vi "AT Command Controller.vi"(2 "error in (no error)":errorcluster, 3 "Command List":T3(array[cluster]), 4 "Boolean Input":u32[](array[numeric])) -> (0 "error out":errorcluster)   [LabVIEW 2018]
uses:
  States.ctl
  Buttons.ctl
  Swerve Drive/Vision Mode.ctl
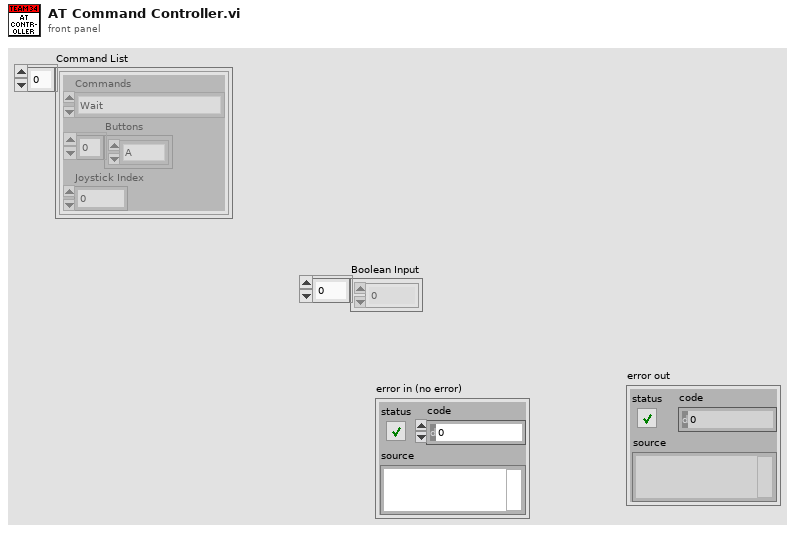
[diagram p1: front panel]
types:
  T1 = typedef "States.ctl" = enum16{"Wait", "Stop", "Limelight Follow", "NavX Reset", "Calibrate Wheels", "Pivot Forward", "Pivot Backward", "Flywheel Forward", "Flywheel Reverse", "FlyDrive Close", "FlyDrive Open", "Pivot Setpoint 0", "Pivot Setpoint 45", "Pivot Setpoint 90", "Low Goal", "Mid Goal", "High Goal", "Low Hatch", "Mid Hatch", "High Hatch", "Vision Track", "Hold Mode"}
  T2 = typedef "Buttons.ctl" = enum16{"A", "B", "X", "Y", "LB", "RB", "Back", "Start", "LS", "RS"}
  T3 = cluster{"Commands":T1, "Buttons":T2[], "Joystick Index":i32}[]
  T4 = typedef "Vision Mode.ctl" = enum16{"Track", "Keep Range", "Follow", "Stop"}
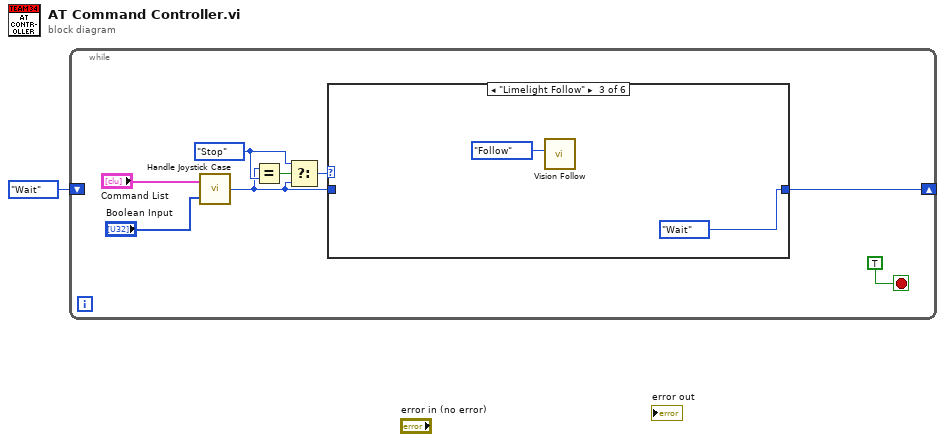
[diagram p0: block diagram]
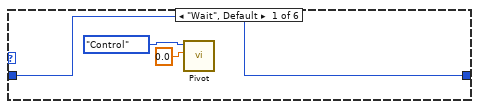
[diagram p2: hidden frame]
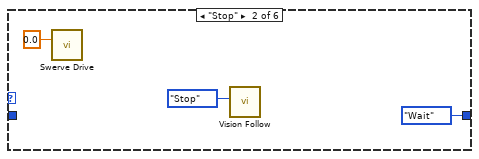
[diagram p3: hidden frame]
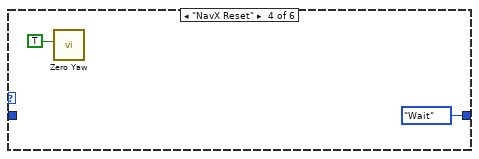
[diagram p4: hidden frame]
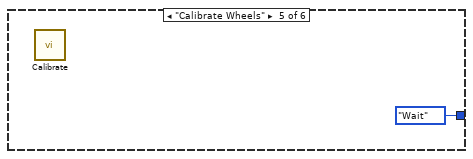
[diagram p5: hidden frame]
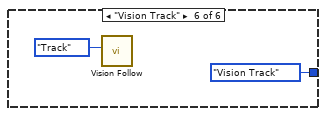
[diagram p6: hidden frame]
diagram:
  n1 = while {
    shift-right: [w4] -> _
    shift-left: States."Wait" ("Commands") -> [_]
    stop <- TRUE stop-if-true
    w6 = States."Stop" ("y")
    n2 = call "Handle Joystick Case.vi"("Boolean Input"="Boolean Input", "Command List"="Command List") -> ("Commands"=w3:T1)
    n3 = Equal?(x=w3, y=w6) -> (x = y?=w7:bool)
    n4 = Select(t=w6, s=w7, f=w3) -> (s? t:f=w5:T1)
    n5 = case shown="\"Limelight Follow\"" w5 {
      tunnel: [w12 States."Wait" ("f") States."Wait" ("f") States."Wait" ("Commands") States."Wait" ("Commands") States."Vision Track" ("Commands")] -> w4
      tunnel: w3 -> [w12 _ _ _ _ _]
      frame "Wait", Default {
        n6 = call "Pivot.vi"("Output"=0.0, "Enum"=enum16{"SetPoint", "Open", "Control"}."Control") -> ()  [unwired: 10 in]
      }
      frame "Stop" {
        n7 = call "Swerve Drive.vi"("Y"=0.0 ("X")) -> ()  [unwired: 10 in, 5 out]
        n8 = call "Vision Follow.vi"("t"=Vision_Mode."Stop") -> ()  [unwired: 11 in]
      }
      frame "Limelight Follow" {
        n9 = call "Vision Follow.vi"("t"=Vision_Mode."Follow") -> ()  [unwired: 11 in]
      }
      frame "NavX Reset" {
        n10 = call <vilib>:"Zero Yaw.vi"("Zero"=TRUE) -> ()  [unwired: 11 in]
      }
      frame "Calibrate Wheels" {
        n11 = call "Calibrate.vi"() -> ()  [unwired: 12 in]
      }
      frame "Vision Track" {
        n12 = call "Vision Follow.vi"("t"=Vision_Mode."Track") -> ()  [unwired: 11 in]
      }
    }
  }
